vi "engenharia.vi"() -> ()   [LabVIEW 2018]
uses:
  Global_Telescopio.vi
panel:
  in  "Case Constant\n(See Context Help)":bool=TRUE
  out "Numeric":i32
  out "Resposta ACK 3":string
  out "String Enviado 3":string
  in  "Recepção":bool
  out "E_Down":bool
  out "W_Down":bool
  out "Base_Limit":bool
  out "DEC_Mesh":bool
  out "RA_Mesh":bool
  out "Inclin_Limite":bool
  out "W_Limite":bool
  out "E_Limite":bool
  out "Leste/Oeste":bool
  out "Chave Power":bool
  out "Vel Zero":bool
  out "Tracking":bool
  out "Embreagem":bool
  out "Indexer":bool
  out "Invrsor":bool
  in  "Tab Control":enum32{"POS.TELESC", "Page 2"}(tab)
  in  "PORTA":refnum<visa-resource-name>="COM12"
  in  "Vel DEC":i32
  in  "Vel AH":i32
  in  "D 2":dbl=4.21 format="%04.1f"
  in  "D 1":i32=32 min=0 max=59
  in  "D 0":i32=-23 min=-103 max=60 format="%#_0f"
  in  "H 2":dbl min=0.0 max=59.99 format="%05.2f"
  in  "H 1":i32 min=0 max=59
  in  "H 0":i32 min=-6 max=6 format="%#_0f"
  out "Resposta ACK 2":string
  out "String Enviado 2":string
  out "Resposta ACK":string
  out "String Enviado":string
  in  "SEND":bool
  in  "GO":bool
  in  "COMANDO":string="AH PROG STATUS"
  in  "SETUP":bool
  out "String":string="BLABLABLABLABLA DA"
  out "Web Server:HTTP Port":u16
  out "Web Server:Server Active":bool
  out "Dados do Computador Remoto Conectado":T1(array[cluster])
  out "Controller Rem/Loc":i32
  in  "ENGENHARIA":bool
  # "Status Information"
  # "Hardware Limits"
  # "Tela Engenharia"
  # "SOMENTE TESTES. NADA AQUI ESTÁ FUNCIONANDO"
  # "Testa Comunicação ENET"
  # "SOMENTE TESTES. NADA AQUI ESTÁ FUNCIONANDO"
  # "ENVIAR PARA O RA(AH) PARA O ENET 192.168.1.4 PORTA 1"
  # "Hour Angle"
  # ":"
  # ":"
  # "AH PROG PARAR"
  # "ALTERADO 14/09/2016"
  # "COM 12 --> AH\nCOM 14 --> CUP\nCOM 15 --> DEC\nCOM 16 --> TUBO"
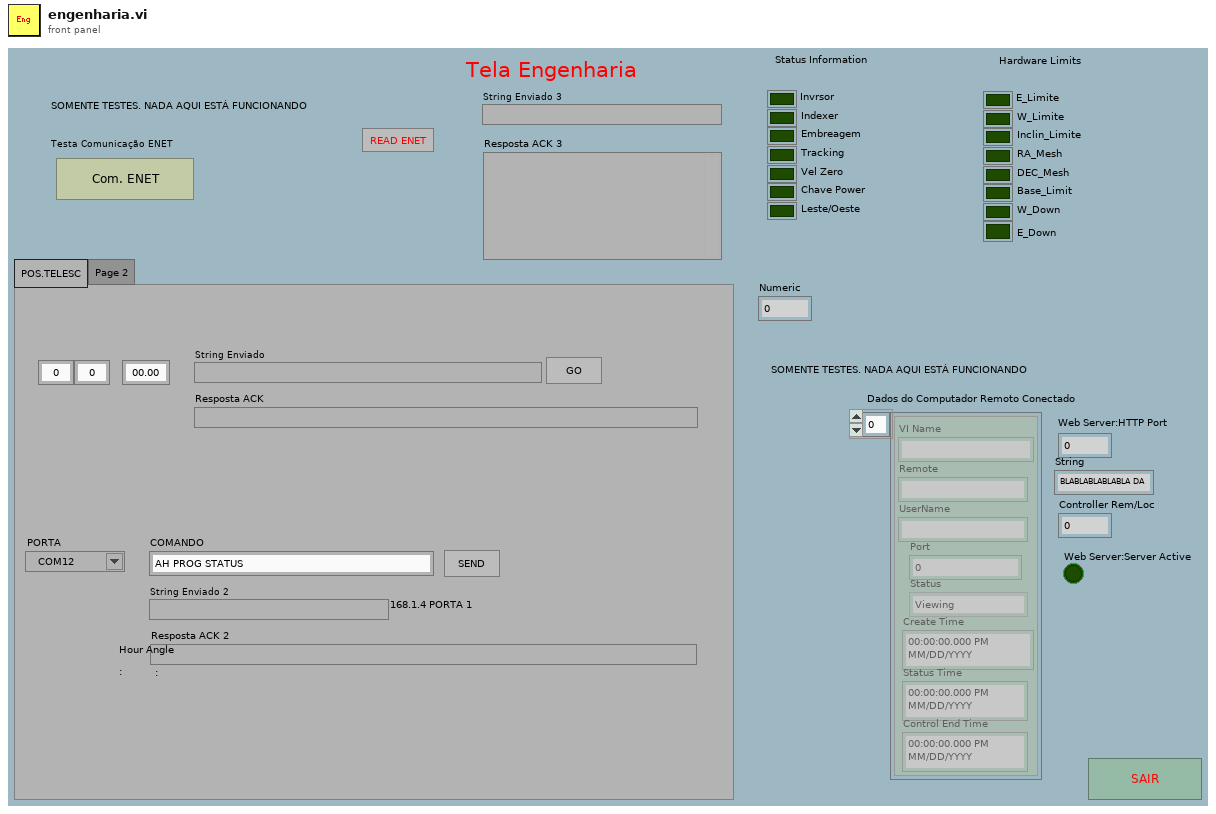
[diagram p1: front panel]
types:
  T1 = cluster{"VI Name":string, "Remote":string, "UserName":string, "Port":i32, "Status":enum32{"Viewing", "Waiting For Control", "Controlling"}, "Create Time":timestamp, "Status Time":timestamp, "Control End Time":timestamp}[]
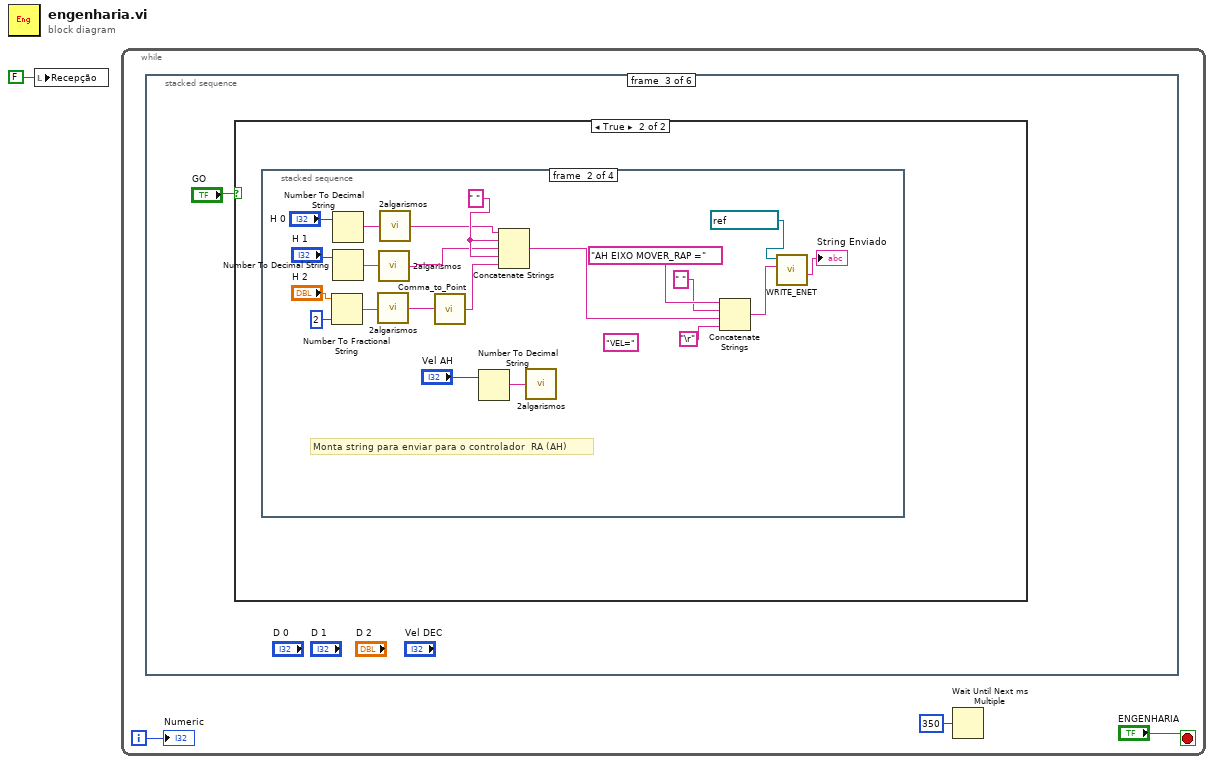
[diagram p0: block diagram]
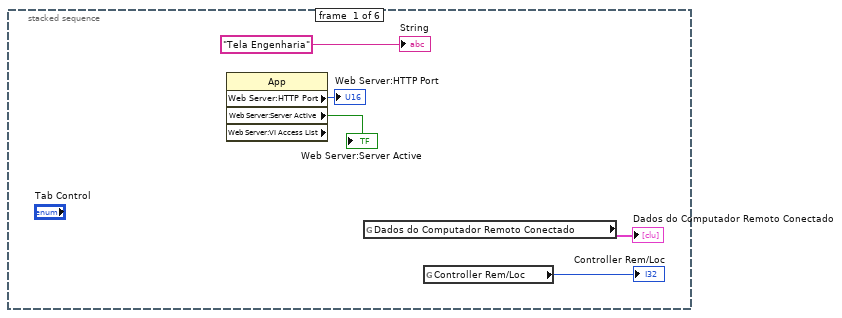
[diagram p2: hidden frame]
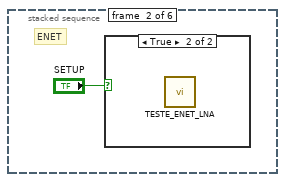
[diagram p3: hidden frame]
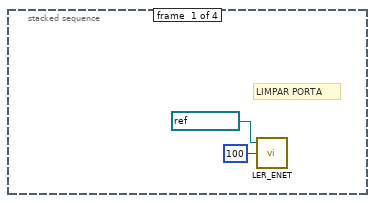
[diagram p6: hidden frame]
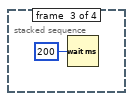
[diagram p7: hidden frame]
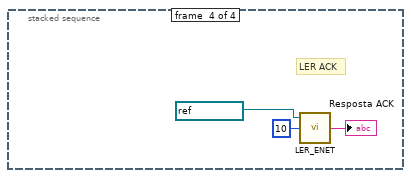
[diagram p8: hidden frame]
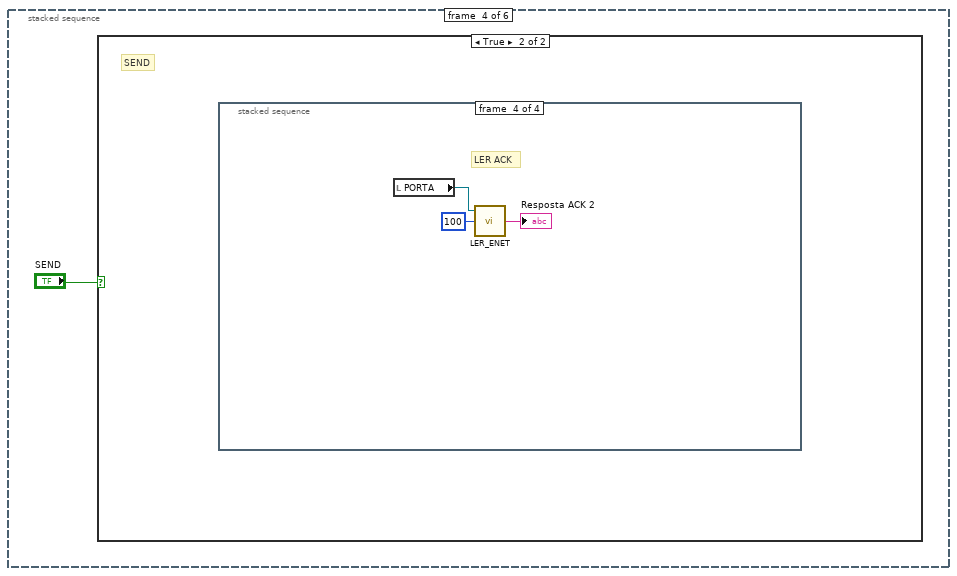
[diagram p9: hidden frame]
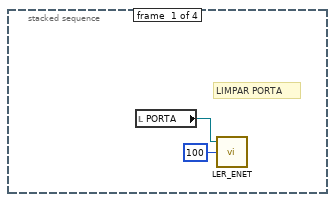
[diagram p11: hidden frame]
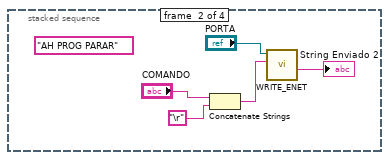
[diagram p12: hidden frame]
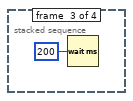
[diagram p13: hidden frame]
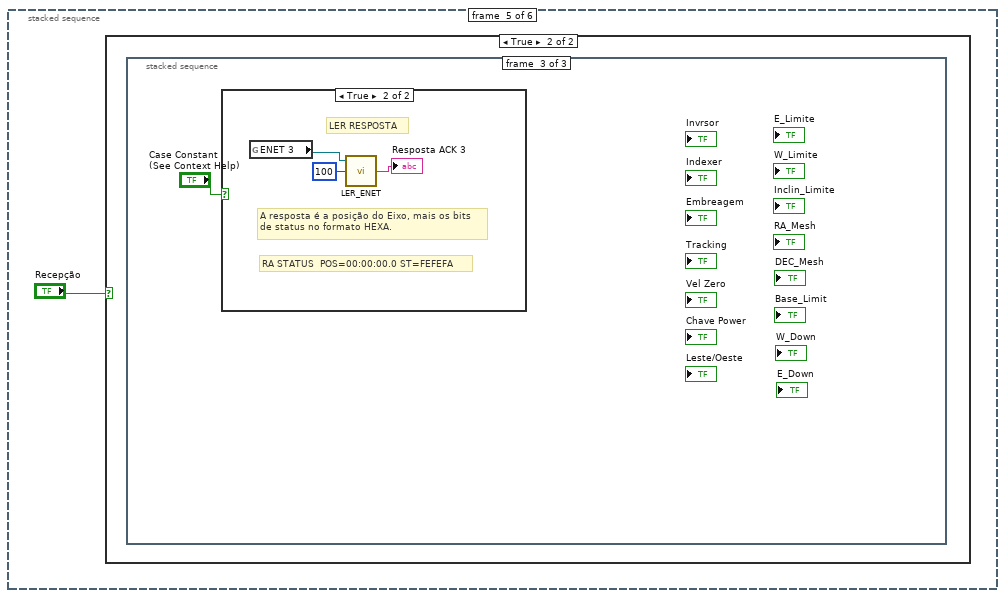
[diagram p14: hidden frame]
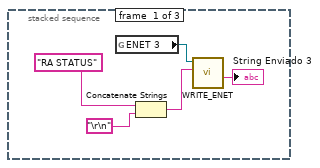
[diagram p16: hidden frame]
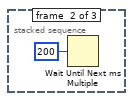
[diagram p17: hidden frame]
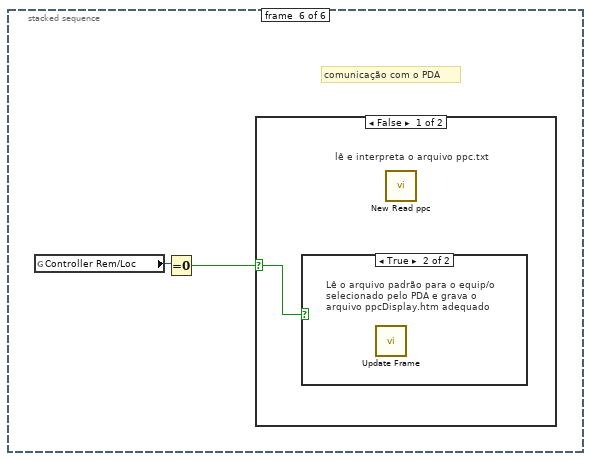
[diagram p19: hidden frame]
diagram:
  n1 = local write "Recepção"(FALSE ("Recepção")) -> ()
  n2 = while {
    i -> [w2]
    stop <- "ENGENHARIA" stop-if-true
    n3 = stacked-sequence {
      frame #0 {
        n4 = property class="App" props=["Web Server:HTTP Port", "Web Server:Server Active", "Web Server:VI Access List"]() -> ("Web Server:HTTP Port"=→"Web Server:HTTP Port":u16, "Web Server:Server Active"=→"Web Server:Server Active":bool)  [unwired: 2 in, 3 out]
        n5 = global read "Global_Telescopio.vi" "Dados do Computador Remoto Conectado"() -> (→"Dados do Computador Remoto Conectado":T1)
        n6 = global read "Global_Telescopio.vi" "Controller Rem/Loc"() -> (→"Controller Rem/Loc":i32)
        "String" <- "Tela Engenharia"
      }
      frame #1 {
        # "ENET"
        n7 = case shown="True" "SETUP" {
          frame False {
          }
          frame True {
            n8 = call "TESTE_ENET_LNA.vi"() -> ()  [unwired: 1 in]
          }
        }
      }
      frame #2 {
        n9 = case shown="True" "GO" {
          frame False {
          }
          frame True {
            n10 = stacked-sequence {
              frame #0 {
                # "LIMPAR PORTA"
                n11 = call "LER_ENET.vi"("Num de Bytes a Ser lido"=u32 100, "LNA VISA resource name"=refnum<visa-resource-name> "COM12" ("PORTA")) -> ()  [unwired: 1 in, 3 out]
              }
              frame #1 {
                w28 = " " ("string")
                (unwired) "VEL=" ("String a ser Enviado")
                # "Monta string para enviar para o controlador  RA (AH)"
                n12 = Number To Fractional String(number="H 2", precision (6)=i16 2) -> (F-format string=w21:string)  [unwired: 2 in]
                n13 = Number To Decimal String(number="H 0") -> (decimal integer string=w24:string)  [unwired: 1 in]
                n14 = Number To Decimal String(number="H 1") -> (decimal integer string=w25:string)  [unwired: 1 in]
                n15 = call "2algarismos.vi"("entrada"=w21) -> ("saida"=w20:string)
                n16 = call "2algarismos.vi"("entrada"=w25) -> ("saida"=w22:string)
                n17 = call "2algarismos.vi"("entrada"=w24) -> ("saida"=w23:string)
                n18 = call "Comma_to_Point.vi"("Lat_A"=w20) -> ("Saída"=w27:string)
                n19 = Number To Decimal String(number="Vel AH") -> (decimal integer string=w19:string)  [unwired: 1 in]
                n20 = Concatenate Strings(w23, w28, w22, w28, w27) -> (w17:string)
                n21 = call "2algarismos.vi"("entrada"=w19) -> ()  [unwired: 1 out]
                n22 = Concatenate Strings("AH EIXO MOVER_RAP =", " ", w17, "\r") -> (w32:string)
                n23 = call "WRITE_ENET.vi"("String a ser Enviado"=w32, "LNA VISA session (for class)"=refnum<visa-resource-name> "COM12" ("PORTA")) -> ("String Enviado"=→"String Enviado":string)  [unwired: 3 in, 2 out]
              }
              frame #2 {
                n24 = Wait (ms)(milliseconds to wait=u32 200) -> ()  [unwired: 1 out]
              }
              frame #3 {
                # "LER ACK"
                n25 = call "LER_ENET.vi"("Num de Bytes a Ser lido"=u32 10, "LNA VISA resource name"=refnum<visa-resource-name> "COM12" ("PORTA")) -> ("String Lida"=→"Resposta ACK":string)  [unwired: 1 in, 2 out]
              }
            }
          }
        }
      }
      frame #3 {
        n26 = case shown="True" "SEND" {
          frame False {
          }
          frame True {
            # "SEND"
            n27 = stacked-sequence {
              frame #0 {
                # "LIMPAR PORTA"
                n28 = local read "PORTA"() -> (w40:refnum<visa-resource-name>)
                n29 = call "LER_ENET.vi"("Num de Bytes a Ser lido"=u32 100, "LNA VISA resource name"=w40) -> ()  [unwired: 1 in, 3 out]
              }
              frame #1 {
                (unwired) "AH PROG PARAR"
                n30 = Concatenate Strings("COMANDO", "\r") -> (w46:string)
                n31 = call "WRITE_ENET.vi"("String a ser Enviado"=w46, "LNA VISA session (for class)"="PORTA") -> ("String Enviado"=→"String Enviado 2":string)  [unwired: 3 in, 2 out]
              }
              frame #2 {
                n32 = Wait (ms)(milliseconds to wait=u32 200) -> ()  [unwired: 1 out]
              }
              frame #3 {
                # "LER ACK"
                n33 = local read "PORTA"() -> (w48:refnum<visa-resource-name>)
                n34 = call "LER_ENET.vi"("Num de Bytes a Ser lido"=u32 100, "LNA VISA resource name"=w48) -> ("String Lida"=→"Resposta ACK 2":string)  [unwired: 1 in, 2 out]
              }
            }
          }
        }
      }
      frame #4 {
        n35 = case shown="True" "Recepção" {
          frame False {
          }
          frame True {
            n36 = stacked-sequence {
              frame #0 {
                n37 = global read "Global_Telescopio.vi" "ENET 3"() -> (w56:refnum<visa-resource-name>)
                n38 = Concatenate Strings("RA STATUS", "\r\n") -> (w55:string)
                n39 = call "WRITE_ENET.vi"("String a ser Enviado"=w55, "LNA VISA session (for class)"=w56) -> ("String Enviado"=→"String Enviado 3":string)  [unwired: 3 in, 2 out]
              }
              frame #1 {
                n40 = Wait Until Next ms Multiple(millisecond multiple=u32 200 ("milliseconds to wait")) -> ()  [unwired: 1 out]
              }
              frame #2 {
                n41 = case shown="True" "Case Constant\n(See Context Help)" {
                  frame False {
                  }
                  frame True {
                    # "RA STATUS  POS=00:00:00.0 ST=FEFEFA"
                    # "A resposta é a posição do Eixo, mais os bits\nde status no formato HEXA."
                    # "LER RESPOSTA"
                    n42 = global read "Global_Telescopio.vi" "ENET 3"() -> (w60:refnum<visa-resource-name>)
                    n43 = call "LER_ENET.vi"("Num de Bytes a Ser lido"=u32 100, "LNA VISA resource name"=w60) -> ("String Lida"=→"Resposta ACK 3":string)  [unwired: 1 in, 2 out]
                  }
                }
              }
            }
          }
        }
      }
      frame #5 {
        # "comunicação com o PDA"
        n44 = global read "Global_Telescopio.vi" "Controller Rem/Loc"() -> (w63:i32)
        n45 = Equal To 0?(x=w63) -> (x = 0?=w62:bool)
        n46 = case shown="False" w62 {
          selector: w62 -> [w64 _]
          frame False {
            # "lê e interpreta o arquivo ppc.txt"
            n47 = case shown="True" w64 {
              frame False {
              }
              frame True {
                # "Lê o arquivo padrão para o equip/o\nselecionado pelo PDA e grava o\narquivo ppcDisplay.htm adequado"
                n48 = call "Update Frame.vi"() -> ()  [unwired: 2 in, 4 out]
              }
            }
            n49 = call "New Read ppc.vi"() -> ()  [unwired: 1 in]
          }
          frame True {
          }
        }
      }
    }
    n50 = Wait Until Next ms Multiple(millisecond multiple=u32 350) -> ()  [unwired: 1 out]
    "Numeric" <- w2
  }
